vi "setDelay.vi"(8 "error in (no error)":errorcluster, 9 "Rate (ps/s)":dbl, 10 "Delay (ps)":dbl, 11 "Instrument.Delay in":refnum<class "Instrument.DelayLine.lvclass">) -> (0 "error out":errorcluster, 3 "Instrument.Delay out":refnum<class "Instrument.DelayLine.lvclass">)   [LabVIEW 2019, in "Instrument.DelayLine.lvclass"]
uses:
  Instrument.DelayLine.lvclass
  Typedefs/DelayLine.setDelay--cluster.ctl
  Typedefs/DelayLine.Commands--Enum.ctl
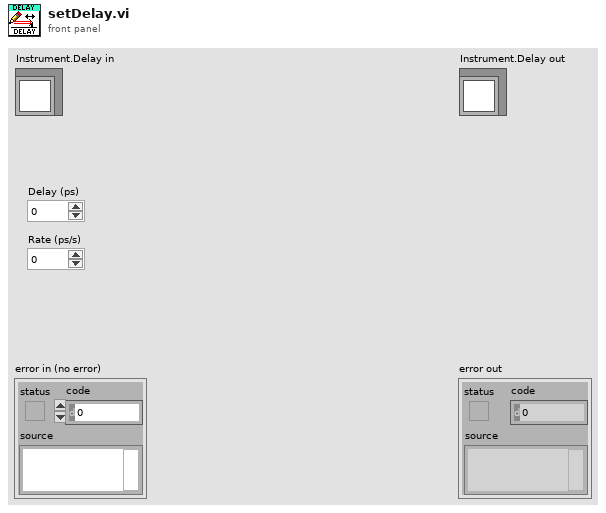
[diagram p1: front panel]
types:
  T1 = typedef "Instrument.DelayLine.lvclass/DelayLine.Commands--Enum.ctl" = enum16{"getDelay", "setDelay"}
  T2 = typedef "Instrument.DelayLine.lvclass/DelayLine.setDelay--cluster.ctl" = cluster{"delay":dbl, "rate":dbl}
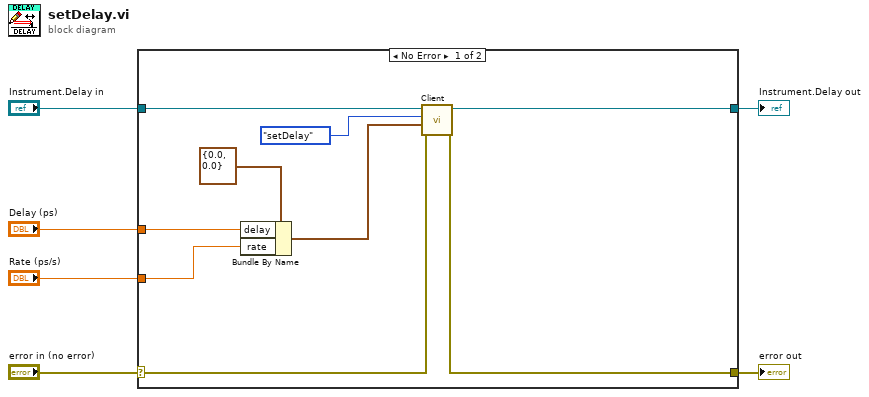
[diagram p0: block diagram]
diagram:
  n1 = case shown="No Error" "error in (no error)" {
    selector: "error in (no error)" -> [w7 w17]
    tunnel: [w14 w17] -> w5
    tunnel: [w15 w16] -> w3
    tunnel: "Instrument.Delay in" -> [w8 w16]
    tunnel: "Delay (ps)" -> [w12 _]
    tunnel: "Rate (ps/s)" -> [w11 _]
    frame No Error {
      n2 = Bundle By Name(cluster=T2 {"delay"=0.0, "rate"=0.0} ("setDelay"), "delay"=w12, "rate"=w11) -> (w10:T2)
      n3 = call-dynamic "Client.vi"("error in (no error)"=w7, "Data in"=w10, "Command in"=DelayLine.Commands--Enum."setDelay" ("command"), "Instrument in"=w8) -> ("error out"=w14:errorcluster, "Instrument out"=w15:refnum<class "Instrument.DelayLine.lvclass">)  [unwired: 4 in, 2 out]
    }
    frame Error {
    }
  }
  "error out" <- w5
  "Instrument.Delay out" <- w3
